vi "scriptWMFSubVI.vi"(8 "error in (no error)":errorcluster, 9 "props cluster":T1, 10 "path":path, 11 "subVI in":refnum<vi>) -> (0 "error out":errorcluster, 1 "props cluster out":T1, 2 "subVI out":refnum<vi>, 3 "VI out":refnum<vi>)   [LabVIEW 2017]
uses:
  <vilib>/express/express shared/propPageData.ctl
  <vilib>/_script/New VI Object TypeDefs/NewVIObject_LVRelativePositionTypeDef.ctl
  <vilib>/_script/New VI Object TypeDefs/NewVIObject_LVRelativeDirectionTypeDef.ctl
  <vilib>/Utility/miscctls.llb/LVPoint32TypeDef.ctl
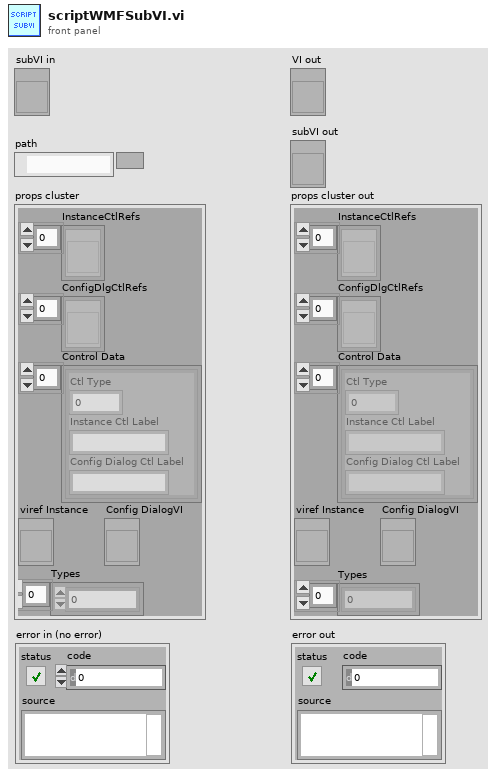
[diagram p1: front panel]
types:
  T1 = typedef "propPageData.ctl" = cluster{"InstanceCtlRefs":refnum<vi>[], "ConfigDlgCtlRefs":refnum<vi>[], "Control Data":cluster{"Ctl Type":u16, "Instance Ctl Label":string, "Config Dialog Ctl Label":string}[], "viref Instance":refnum<vi>, "Types":i32[], "Config DialogVI":refnum<vi>}
  T2 = typedef "NewVIObject_LVRelativeDirectionTypeDef.ctl" = enum32{"Right", "Left", "Top", "Bottom", "Top Right", "Top Left", "Bottom Right", "Bottom Left"}
  T3 = typedef "NewVIObject_LVRelativePositionTypeDef.ctl" = cluster{"Refnum":refnum<vi>, "Relative Direction":T2, "Point32":T4}
  T4 = typedef "LVPoint32TypeDef.ctl" = cluster{"Horizontal":i32, "Vertical":i32}
  T5 = typedef "LVFontTypeDef.ctl" = cluster{"Font Name":string, "Size":u16, "Bold":bool, "Italic":bool, "Underline":bool, "Strikeout":bool, "Color":u32}
  T6 = typedef "LVSelectionTypeDef.ctl" = cluster{"Selection Start":u32, "Selection End":u32}
  T7 = typedef "LVTextColorsTypeDef.ctl" = cluster{"Text Color":u32, "Background Color":u32}
  T8 = enum16{"None", "Stacked", "Clockwise", "Counterclockwise"}
  T9 = cluster{"Ctl Type":u16, "Instance Ctl Label":string, "Config Dialog Ctl Label":string}[]
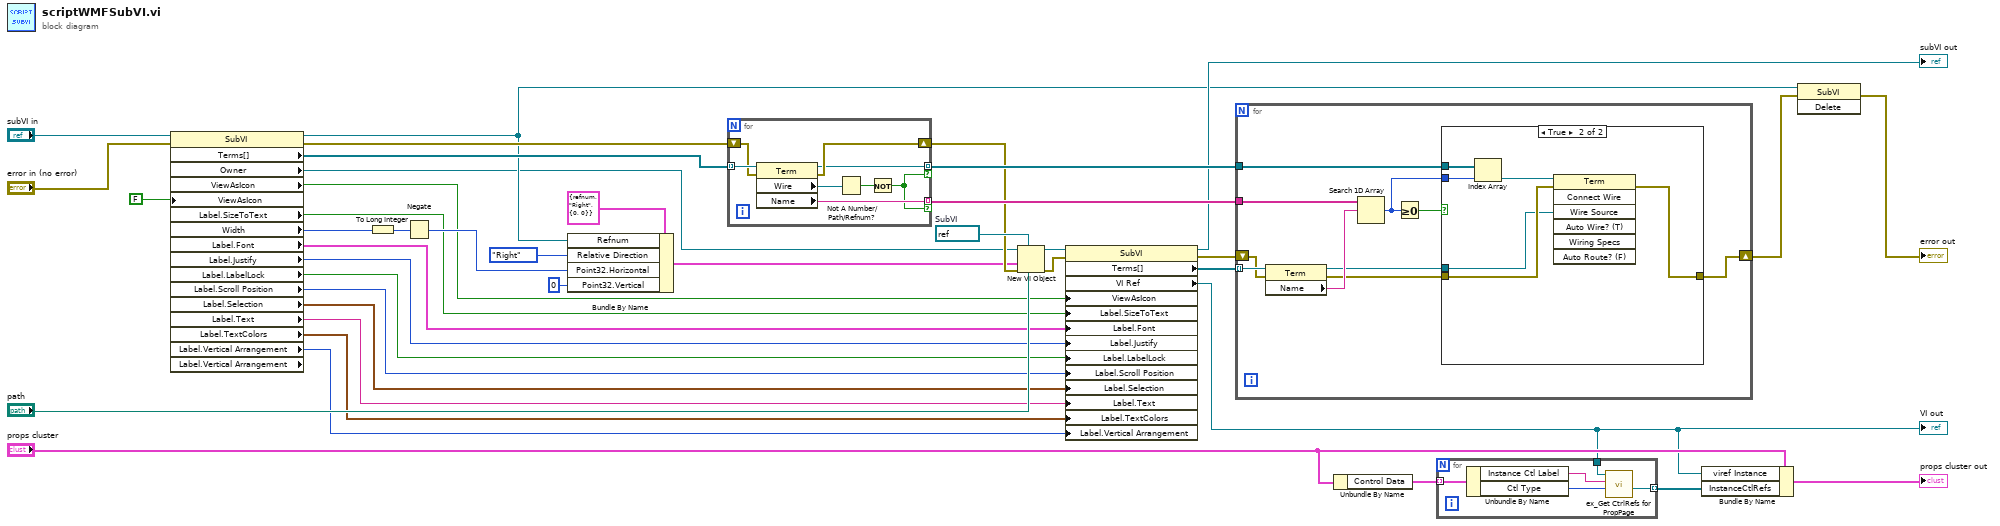
[diagram p0: block diagram]
diagram:
  w40 = refnum<vi> refnum  # SubVI
  n1 = property class="SubVI" props=["Terms[]", "Owner", "ViewAsIcon", "ViewAsIcon", "Label", "SizeToText", "Width", "Label", "Font", "Label", "Justify", "Label", "LabelLock", "Label", "Scroll Position", "Label", "Selection", "Label", "Text", "Label", "TextColors", "Label", "Vertical Arrangement", "Label", "Vertical Arrangement"](reference="subVI in", error in="error in (no error)", "ViewAsIcon"=FALSE ("View As Icon")) -> (reference out=w20:refnum<vi>, error out=w23:errorcluster, "Terms[]"=w39:refnum<vi>[], "Owner"=w17:refnum<vi>, "ViewAsIcon"=w5:bool, "Label.SizeToText"=w1:bool, "Width"=w8:u32, "Label.Font"=w16:T5, "Label.Justify"=w15:enum16{"Left", "Center", "Right"}, "Label.LabelLock"=w14:bool, "Label.Scroll Position"=w13:u32, "Label.Selection"=w12:T6, "Label.Text"=w11:string, "Label.TextColors"=w10:T7, "Label.Vertical Arrangement"=w9:T8)  [unwired: 1 out]
  n2 = To Long Integer(number=w8) -> (32bit integer=w18:i32)
  n3 = Negate(x=w18) -> (-x=w7:i32)
  n4 = Bundle By Name(cluster=T3 {"Refnum"=refnum, "Relative Direction"=enum."Right", "Point32"={"Horizontal"=0, "Vertical"=0}} ("Relative Position"), "Refnum"=w20, "Relative Direction"=NewVIObject_LVRelativeDirectionTypeDef."Right", "Point32.Horizontal"=w7, "Point32.Vertical"=0) -> (w21:T3)
  n5 = for {
    tunnel: w39 -> [w49] mode=indexing
    tunnel: [w42] -> w35 mode=indexing if=w43
    tunnel: [w48] -> w34 mode=indexing if=w43
    shift-right: [w44] -> w28
    shift-left: w23 -> [w45]
    n6 = property class="Term"(reference=w49, error in=w45) -> (reference out=w42:refnum<vi>, error out=w44:errorcluster, "Wire"=w47:refnum<vi>, "Name"=w48:string)
    n7 = Not A Number/Path/Refnum?(number/path/refnum=w47) -> (NaN/Path/Refnum?=w46:bool)
    n8 = Not(x=w46) -> (.not. x?=w43:bool)
  }
  n9 = New VI Object(vi object class=w40, owner refnum=w17, position/next to=w21, 6:"path", 8:w28) -> (object refnum=w24:refnum<vi>, 0:w25:errorcluster)  [unwired: 3 in]
  n10 = property class="SubVI"(reference=w24, error in=w25, "ViewAsIcon"=w5, "Label.SizeToText"=w1, "Label.Font"=w16, "Label.Justify"=w15, "Label.LabelLock"=w14, "Label.Scroll Position"=w13, "Label.Selection"=w12, "Label.Text"=w11, "Label.TextColors"=w10, "Label.Vertical Arrangement"=w9) -> (reference out=→"subVI out":refnum<vi>, error out=w33:errorcluster, "Terms[]"=w36:refnum<vi>[], "VI Ref"=w2:refnum<vi>)
  "VI out" <- w2
  n11 = for {
    tunnel: w36 -> [w59] mode=indexing
    tunnel: w35 -> [w55]
    tunnel: w34 -> [w58]
    shift-right: [w50] -> w27
    shift-left: w33 -> [w52]
    n12 = property class="Term"(reference=w59, error in=w52) -> (reference out=w53:refnum<vi>, error out=w51:errorcluster, "Name"=w57:string)
    n13 = Search 1D Array(1D array=w58, element=w57) -> (index of element=w54:i32)  [unwired: 1 in]
    n14 = Greater Or Equal To 0?(x=w54) -> (x >= 0?=w56:bool)
    n15 = case shown="True" w56 {
      tunnel: w55 -> [_ w66]
      tunnel: w54 -> [_ w65]
      tunnel: w53 -> [_ w61]
      tunnel: w51 -> [w60 w62]
      tunnel: [w60 w64] -> w50
      frame False {
      }
      frame True {
        n16 = Index Array(array=w66, index=w65) -> (element=w63:refnum<vi>)
        n17 = invoke class="Term" method="Connect Wire"(reference=w63, error in=w62, "Wire Source"=w61) -> (error out=w64:errorcluster)  [unwired: 4 in, 6 out]
      }
    }
  }
  n18 = Unbundle By Name("props cluster") -> ("Control Data"=w32:T9)
  n19 = for {
    tunnel: w2 -> [w71]
    tunnel: w32 -> [w70] mode=indexing
    tunnel: [w69] -> w3 mode=indexing
    n20 = Unbundle By Name(w70) -> ("Instance Ctl Label"=w67:string, "Ctl Type"=w68:u16)
    n21 = call <vilib>:"ex_Get CtrlRefs for PropPage.vi"("Ctl Type"=w68, "Object Name"=w67, "Express VI"=w71) -> ("Output Reference"=w69:refnum<vi>)  [unwired: 6 in, 2 out]
  }
  n22 = Bundle By Name(cluster="props cluster", "viref Instance"=w2, "InstanceCtlRefs"=w3) -> (→"props cluster out":T1)
  n23 = invoke class="SubVI" method="Delete"(reference=w20, error in=w27) -> (error out=→"error out":errorcluster)  [unwired: 1 in, 2 out]
